vi "Wave2D_Cal U_Apply BC_X.vi"(8 "x length":i32, 9 "End X Value":dbl[](array[numeric]), 10 "Start X Value":dbl[](array[numeric]), 11 "U In":dbl[][](array[numeric])) -> (3 "U Out":dbl[][](array[numeric]))   [LabVIEW 2020, in "NI_PDE.lvlib"]
uses:
  <vilib>/gmath/NI_PDE.lvlib
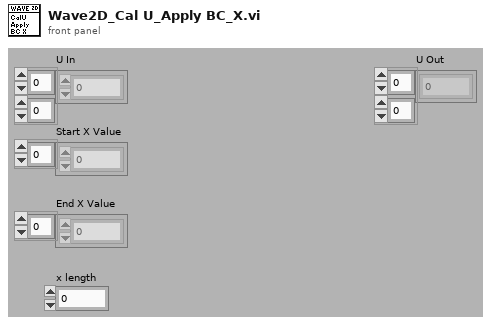
[diagram p1: front panel]
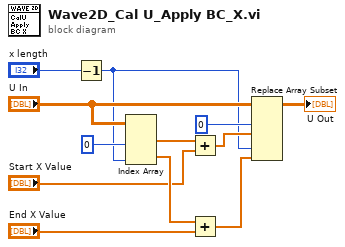
[diagram p0: block diagram]
diagram:
  n1 = Decrement(x="x length") -> (x-1=w4:i32)
  n2 = Index Array(array="U In", index (col) #1=0 ("disabled index (col)"), index (col) #2=w4) -> (element #1=w12:dbl[], element #2=w11:dbl[])  [unwired: 2 in]
  n3 = Add(x=w12, y="Start X Value") -> (x+y=w10:dbl[])
  n4 = Add(x=w11, y="End X Value") -> (x+y=w9:dbl[])
  n5 = Replace Array Subset(array="U In", new element #1=w10, index (col) #1=0 ("disabled index (col)"), new element #2=w9, index (col) #2=w4) -> (→"U Out":dbl[][])  [unwired: 2 in]
